vi "CC Edit Hardware Type.vi"(8 "error in (no error)":errorcluster, 11 "Device":T1) -> (0 "error out":errorcluster, 1 "cancelled?":bool, 3 "Device out":T1)   [LabVIEW 2021]
uses:
  typedefs/CC cluster Device Index.ctl
panel:
  in  "Instances":string[](array[string])
  in  "Cancel":bool
  in  "Ok":bool
  in  "Hardware Type":string
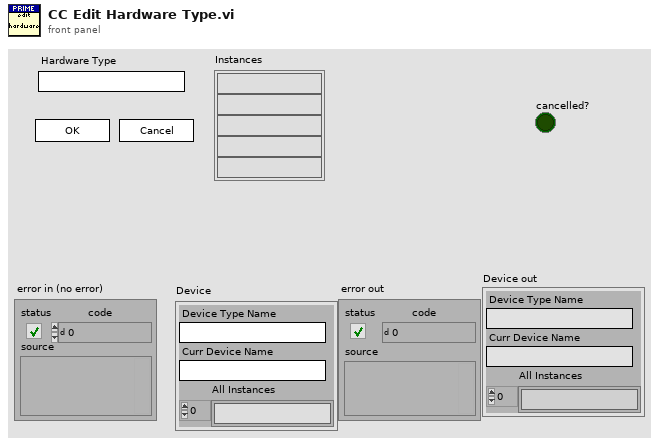
[diagram p1: front panel]
types:
  T1 = typedef "CC cluster Device Index.ctl" = cluster{"Device Type Name":string, "Curr Device Name":string, "All Instances":string[]}
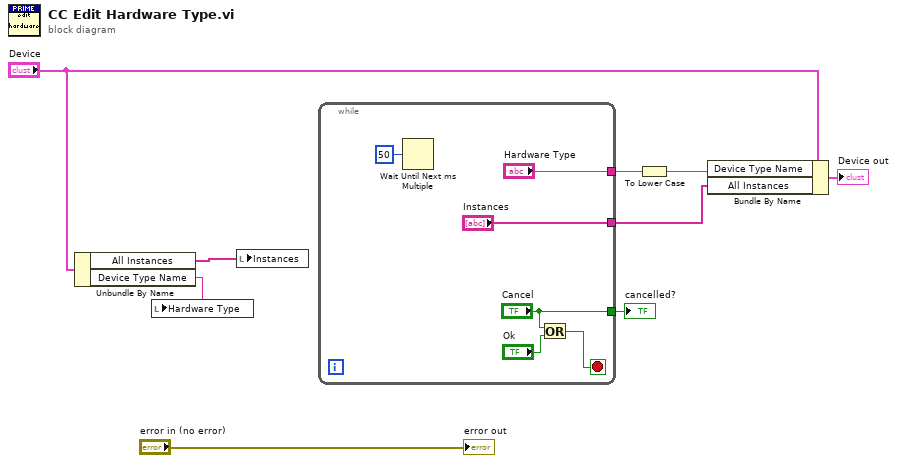
[diagram p0: block diagram]
diagram:
  n1 = Unbundle By Name("Device") -> ("All Instances"=w2:string[], "Device Type Name"=w7:string)
  n2 = local write "Hardware Type"(w7) -> ()
  n3 = local write "Instances"(w2) -> ()
  n4 = while {
    tunnel: ["Instances"] -> w4
    tunnel: ["Hardware Type"] -> w5
    tunnel: ["Cancel"] -> w8
    stop <- w13 stop-if-true
    n5 = Wait Until Next ms Multiple(millisecond multiple=u32 50) -> ()  [unwired: 1 out]
    n6 = Or(x="Cancel", y="Ok") -> (x .or. y?=w13:bool)
  }
  "cancelled?" <- w8
  n7 = To Lower Case(string=w5) -> (all lower case string=w1:string)
  n8 = Bundle By Name(cluster="Device", "Device Type Name"=w1, "All Instances"=w4) -> (→"Device out":T1)
  "error out" <- "error in (no error)"
